vi "Valve Globals.vi"() -> ()   [LabVIEW 2018]
panel:
  out "Turbo pump time":dbl=7200.0
  out "Roughing pump time":dbl=300.0
  out "Valves 1 and 2 vent time":dbl=40.0
  out "Valves 5 and 7 vent time":dbl=10.0
  out "Valve 6 vent time":dbl=10.0
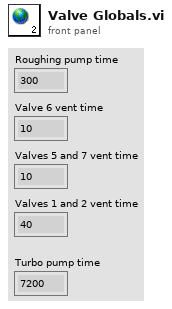
[diagram p1: front panel]
diagram:
